vi "provide_OME_data.vi"(6 "image ID":string, 8 "error in (no error)":errorcluster, 9 "structuredAttribute string in":string, 10 "OME element in":refnum<class "XMLElement.lvclass">, 11 "ScanHeadDL090202 in":refnum<class "ScanHeadDL090202.lvclass">) -> (0 "error out":errorcluster, 1 "structuredAttribute string out":string, 2 "OME element out":refnum<class "XMLElement.lvclass">, 3 "ScanHeadDL090202 out":refnum<class "ScanHeadDL090202.lvclass">)   [LabVIEW 2010, in "ScanHeadDL090202.lvclass"]
uses:
  ScanHeadDL090202.lvclass
  GenericScanHead/GenericScanHead/GenericScanHead.lvclass
  SignalWriter/GenericSignalWriter/GenericSignalWriter/GenericSignalWriter.lvclass
  common/classes/ErrorController/ErrorController/ErrorController.lvclass
  common/classes/XMLElement/XMLElement/XMLElement.lvclass
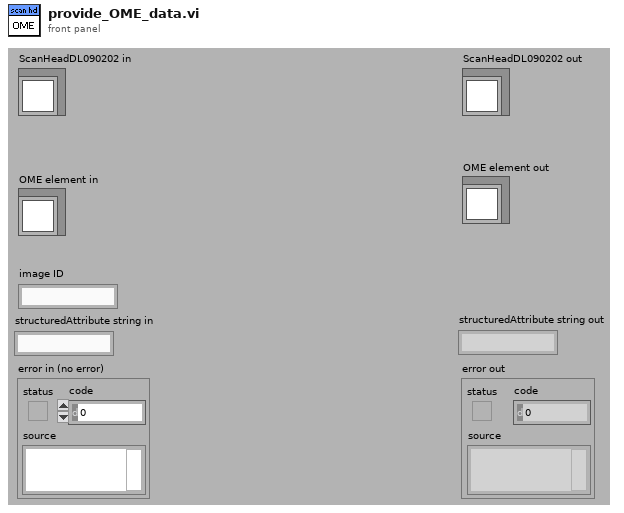
[diagram p1: front panel]
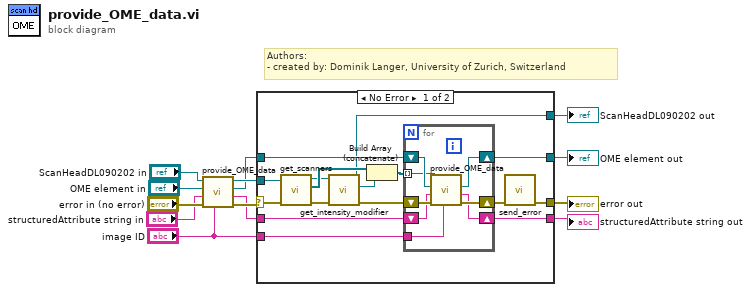
[diagram p0: block diagram]
diagram:
  # "Authors: \n- created by: Dominik Langer, University of Zurich, Switzerland"
  n1 = call-parent "provide_OME_data.vi"("image ID"="image ID", "error in (no error)"="error in (no error)", "structuredAttribute string in"="structuredAttribute string in", "OME element in"="OME element in", "GenericScanHead in"="ScanHeadDL090202 in") -> ("error out"=w10:errorcluster, "structuredAttribute string out"=w2:string, "OME element out"=w8:refnum<class "XMLElement.lvclass">, "GenericScanHead out"=w9:refnum<class "ScanHeadDL090202.lvclass">)  [unwired: 3 in]
  n2 = case shown="No Error" w10 {
    selector: w10 -> [w29 w41]
    tunnel: w9 -> [w28 w39]
    tunnel: w8 -> [w27 w40]
    tunnel: [w16 w41] -> w7
    tunnel: "image ID" -> [w26 _]
    tunnel: [w25 w40] -> w5
    tunnel: [w18 w39] -> w6
    tunnel: w2 -> [w15 w38]
    tunnel: [w14 w38] -> w1
    frame No Error {
      n3 = call-dynamic "get_scanners.vi"("error in (no error)"=w29, "DL090202ScanHead.lvclass in"=w28) -> ("error out"=w24:errorcluster, "scanners"=w20:refnum<class "GenericSignalWriter.lvclass">[], "DL090202ScanHead.lvclass out"=w19:refnum<class "ScanHeadDL090202.lvclass">)  [unwired: 7 in]
      n4 = call-dynamic "get_intensity_modifier.vi"("error in (no error)"=w24, "DL090202ScanHead.lvclass in"=w19) -> ("error out"=w23:errorcluster, "write signals"=w21:refnum<class "GenericSignalWriter.lvclass">, "DL090202ScanHead.lvclass out"=w18:refnum<class "ScanHeadDL090202.lvclass">)  [unwired: 7 in]
      n5 = Build Array (concatenate)(w20, w21) -> (w22:refnum<class "GenericSignalWriter.lvclass">[])
      n6 = for {
        tunnel: w22 -> [w33] mode=indexing
        tunnel: w26 -> [w32]
        shift-right: [w36] -> w17
        shift-left: w23 -> [w37]
        shift-right: [w34] -> w25
        shift-left: w27 -> [w35]
        shift-right: [w30] -> w14
        shift-left: w15 -> [w31]
        n7 = call-dynamic "provide_OME_data.vi"("image ID"=w32, "error in (no error)"=w37, "structuredAttribute string in"=w31, "OME element in"=w35, "GenericPlugin in"=w33) -> ("error out"=w36:errorcluster, "structuredAttribute string out"=w30:string, "OME element out"=w34:refnum<class "XMLElement.lvclass">)  [unwired: 3 in, 1 out]
      }
      n8 = call "send_error.vi"("error in (no error)"=w17) -> ("error out"=w16:errorcluster)  [unwired: 10 in]
    }
    frame Error {
    }
  }
  "error out" <- w7
  "ScanHeadDL090202 out" <- w6
  "OME element out" <- w5
  "structuredAttribute string out" <- w1
